vi "Add Event Reference to maps.vi"(7 "Root Path":string, 8 "Event Type":T1, 9 "Event VIs":refnum<vi>[](array[refnum]), 10 "Tree Map in":T2) -> (2 "Tree Map out":T2)   [LabVIEW 2019, in "Panther Dashboard.lvlib"]
uses:
  Panther Dashboard.lvlib
  <vilib>/National Instruments/Tree Map/Tree Map Data.ctl
  Map Attribute--enum.ctl
  <vilib>/National Instruments/Tree Map/Tree Map.lvlib
  <vilib>/Delacor/Delacor QMH/Libraries/_Scripting Support/Event Type (New)--enum.ctl
  <vilib>/Delacor/Delacor QMH/Libraries/_Scripting Support/dqmh_lib_DQMH Scripting Support.lvlib
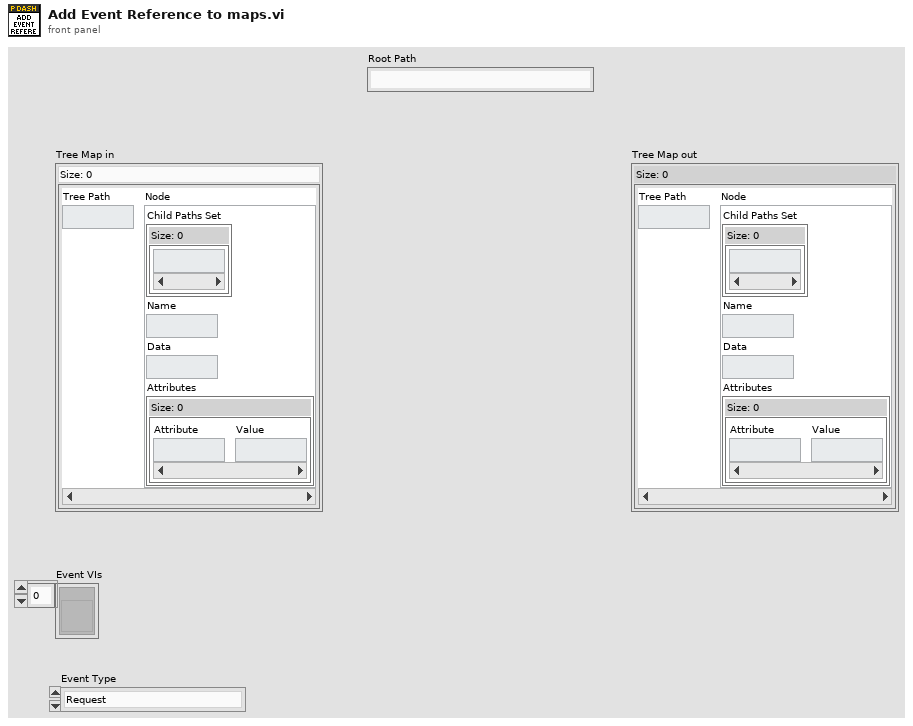
[diagram p1: front panel]
types:
  T1 = typedef "dqmh_lib_DQMH Scripting Support.lvlib/Event Type (New)--enum.ctl" = enum16{"Request", "Broadcast", "Request and Wait for Reply", "Round Trip"}
  T2 = typedef "Tree Map.lvlib/Tree Map Data.ctl" = map{string, cluster{"Child Paths Set":set{string}, "Name":string, "Data":string, "Attributes":map{string, string}}}
  T3 = typedef "Panther Dashboard.lvlib/Map Attribute--enum.ctl" = enum16{"Path", "ModuleType", "Module Description", "Dependency?", "Target"}
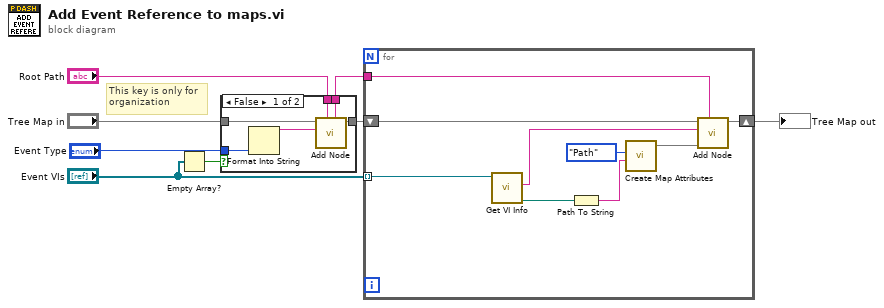
[diagram p0: block diagram]
diagram:
  # "This key is only for\norganization"
  n1 = Empty Array?(array="Event VIs") -> (empty?=w2:bool)
  n2 = case shown="False" w2 {
    tunnel: "Root Path" -> [w13 w16]
    tunnel: [w12 w16] -> w6
    tunnel: "Tree Map in" -> [w11 w15]
    tunnel: [w10 w15] -> w4
    tunnel: "Event Type" -> [w9 _]
    frame False {
      n3 = Format Into String(w9) -> (resulting string=w14:string)  [unwired: 3 in, 1 out]
      n4 = call <vilib>:"Add Node.vi"("Parent Path"=w13, "New Node Name"=w14, "Tree Map In"=w11) -> ("Tree Map Out"=w10:T2, "New Node Path"=w12:string)  [unwired: 6 in, 1 out]
    }
    frame True {
    }
  }
  n5 = for {
    tunnel: w6 -> [w25]
    shift-right: [w23] -> w8
    shift-left: w4 -> [w24]
    tunnel: "Event VIs" -> [w21] mode=indexing
    n6 = call "Get VI Info.vi"("VI in"=w21) -> ("VI Path"=w17:path, "Plain Name"=w22:string)  [unwired: 7 in, 2 out]
    n7 = Path To String(path=w17) -> (string=w18:string)
    n8 = call "Create Map Attributes.vi"("Attribute"=w18, "Map Attribute"=Map_Attribute--enum."Path") -> ("Root Attributes"=w20:map{string, string})  [unwired: 9 in]
    n9 = call <vilib>:"Add Node.vi"("Parent Path"=w25, "Attributes"=w20, "New Node Name"=w22, "Tree Map In"=w24) -> ("Tree Map Out"=w23:T2)  [unwired: 5 in, 2 out]
  }
  "Tree Map out" <- w8
